vi "service_dequeue.vi"(0 "queue":refnum<queue>, 11 "error in":errorcluster) -> (4 "queue out":refnum<queue>, 6 "JSON Tree Out Passthrough":variant, 8 "function name":string, 10 "# elements in queue":i32, 15 "error out":errorcluster)   [LabVIEW 2010]
uses:
  i3-json-1.0.0-10/JSON Parsing/Get Object Parameter Files/Get Object Parameter - String.vi
  i3-json-1.0.0-10/i3-json.lvlib
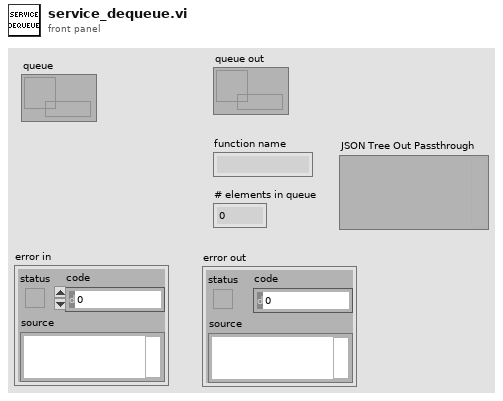
[diagram p1: front panel]
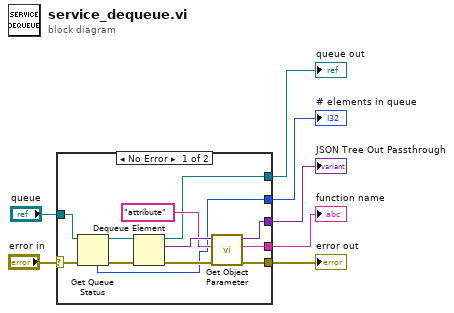
[diagram p0: block diagram]
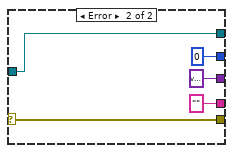
[diagram p2: hidden frame]
diagram:
  n1 = case shown="No Error" "error in" {
    selector: "error in" -> [w13 w22]
    tunnel: "queue" -> [w14 w23]
    tunnel: [w12 0 ("# elements in queue")] -> w5
    tunnel: [w11 w23] -> w4
    tunnel: [w10 "" ("String Value")] -> w3
    tunnel: [w9 w22] -> w2
    tunnel: [w8 variant ("JSON Tree Out Passthrough")] -> w1
    frame No Error {
      n2 = Get Queue Status(queue=w14, error in (no error)=w13) -> (queue out=w19:refnum<queue>, error out=w18:errorcluster, # elements in queue=w12:i32)  [unwired: 1 in, 5 out]
      n3 = Dequeue Element(queue=w19, error in (no error)=w18) -> (queue out=w11:refnum<queue>, element=w17:variant, error out=w15:errorcluster)  [unwired: 1 in, 1 out]
      n4 = call-poly "Get Object Parameter.vi"("error in (no error)"=w15, "Parameter Name"="attribute", "JSON Tree In (JSON Object)"=w17) -> ("error out"=w9:errorcluster, "String Value"=w10:string, "JSON Tree Out Passthrough"=w8:variant)  [unwired: 5 in, 1 out]
    }
    frame Error {
    }
  }
  "# elements in queue" <- w5
  "queue out" <- w4
  "function name" <- w3
  "error out" <- w2
  "JSON Tree Out Passthrough" <- w1
